vi "Update Delta Time.vi"(5 "reinit":bool, 7 "skip":bool, 8 "error in (no error)":errorcluster, 9 "T2":u64, 10 "T1":u64, 11 "Timing in":cluster{"Max":i32, "Min":i32}) -> (0 "error out":errorcluster, 3 "Timing out":cluster{"Max":i32, "Min":i32})   [LabVIEW 2021, in "CIFCoreCommon.lvlib"]
uses:
  CIFCoreCommon.lvlib
  CIFUtilities/CIFClocks/Typedef/Errors.ctl
  Append Error Location.vi
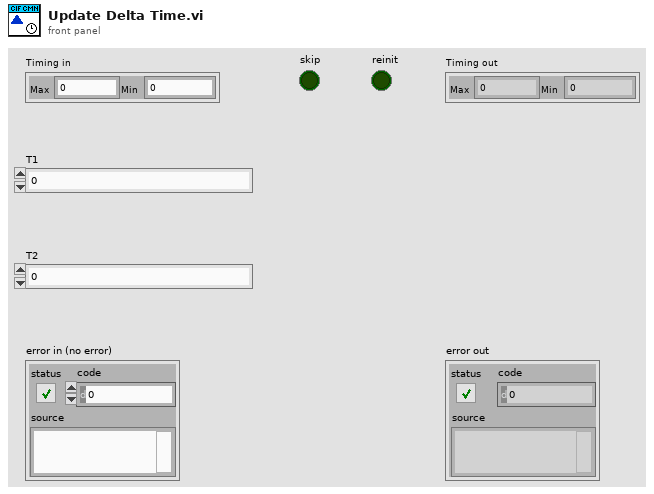
[diagram p1: front panel]
types:
  T1 = typedef "CIFCoreCommon.lvlib/Errors.ctl" = enum16{"Invalid Clock ID", "Long Sleep", "gRPC Server Not Found", "Config Parse", "Timestamp Wrap", "Delayed Execution", "Duplicate Channel", "Missing Channel", "Incorrect Type"}
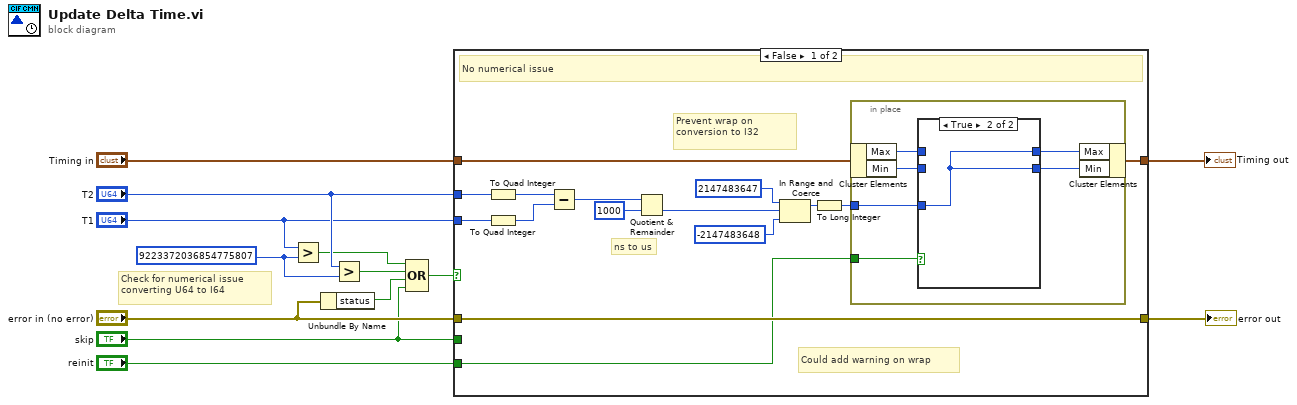
[diagram p0: block diagram]
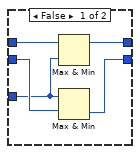
[diagram p2: hidden frame]
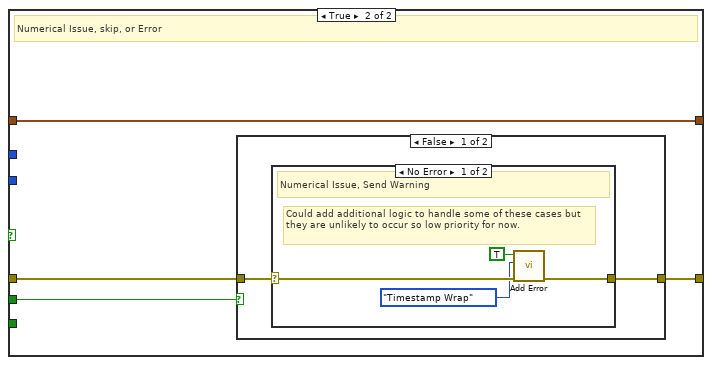
[diagram p3: hidden frame]
diagram:
  w4 = u64 9223372036854775807 ("floor(x/y)")
  # "Check for numerical issue converting U64 to I64"
  n1 = Greater?(x="T1", y=w4) -> (0:w7:bool)
  n2 = Unbundle By Name("error in (no error)") -> ("status"=w3:bool)
  n3 = Greater?(x="T2", y=w4) -> (0:w6:bool)
  n4 = Compound Arithmetic op=OR(w7, w6, w3, "skip") -> (w5:bool)
  n5 = case shown="False" w5 {
    tunnel: "Timing in" -> [w26 w44]
    tunnel: [w25 w44] -> w12
    tunnel: "T2" -> [w24 _]
    tunnel: "T1" -> [w23 _]
    tunnel: "error in (no error)" -> [w22 w43]
    tunnel: [w22 w42] -> w8
    tunnel: "skip" -> [_ w41]
    tunnel: "reinit" -> [w14 _]
    frame False {
      # "ns to us"
      # "Could add warning on wrap"
      # "Prevent wrap on conversion to I32"
      # "No numerical issue"
      n6 = To Quad Integer(1:w24) -> (0:w28:i64)
      n7 = To Quad Integer(1:w23) -> (0:w27:i64)
      n8 = Subtract(x=w28, y=w27) -> (x-y=w17:i64)
      n9 = Quotient & Remainder(x=w17, y=i64 1000) -> (floor(x/y)=w15:i64)  [unwired: 1 out]
      n10 = In Range and Coerce(upper limit=i64 2147483647 ("Min"), x=w15, lower limit=i64 -2147483648 ("Min")) -> (coerced(x)=w21:i64)  [unwired: 1 out]
      n11 = To Long Integer(number=w21) -> (32bit integer=w18:i32)
      n12 = in-place {
        in-place-border: w18 -> [w30]
        in-place-border: w14 -> [w29]
        n13 = in-place-cluster #1(w26) -> ("Max"=w34:i32, "Min"=w32:i32)
        n14 = case shown="True" w29 {
          tunnel: w34 -> [w39 _]
          tunnel: [w38 w40] -> w33
          tunnel: w32 -> [w37 _]
          tunnel: [w36 w40] -> w31
          tunnel: w30 -> [w35 w40]
          frame False {
            n15 = Max & Min(x=w39, y=w35) -> (max(x,y)=w38:i32)  [unwired: 1 out]
            n16 = Max & Min(x=w35, y=w37) -> (min(x,y)=w36:i32)  [unwired: 1 out]
          }
          frame True {
          }
        }
        n17 = in-place-cluster #1("Max"=w33, "Min"=w31) -> (w25:cluster{"Max":i32, "Min":i32})
      }
    }
    frame True {
      # "Numerical Issue, skip, or Error"
      n18 = case shown="False" w41 {
        tunnel: w43 -> [w46 w52]
        tunnel: [w45 w52] -> w42
        frame False {
          n19 = case shown="No Error" w46 {
            selector: w46 -> [w50 w51]
            tunnel: [w49 w51] -> w45
            frame No Error {
              # "Could add additional logic to handle some of these cases but they are unlikely to occur so low priority for now."
              # "Numerical Issue, Send Warning"
              n20 = call "Add Error.vi"("error in (no error)"=w50, "Error"=Errors."Timestamp Wrap", "Insert Error"=TRUE) -> ("error out"=w49:errorcluster)  [unwired: 8 in]
            }
            frame Error {
              # "Error"
            }
          }
        }
        frame True {
          # "Skip logic"
        }
      }
    }
  }
  "Timing out" <- w12
  "error out" <- w8
